vi "Autonomous Independent.vi"   [LabVIEW 2019]
doc: "This VI is called when autonomous begins, and will automatically be terminated when autonomous ends. You can carry out timed or sensor driven robot movement independently without needing to return to the caller."
uses:
  <vilib>/Rock Robotics/WPI/ThirdParty/Phoenix-LabVIEW/Motor Controller/Controls/CTRE_Phoenix_MotorControl_ControlMode.ctl
  <vilib>/Rock Robotics/WPI/Utilities/WPI_GetSetVariantRefNum.vi
  <vilib>/Rock Robotics/Network Tables/NT Read String.vi
  <vilib>/Rock Robotics/Network Tables/NT Write Numeric Array.vi
  <vilib>/Rock Robotics/WPI/RobotDrive/WPI_RobotDriveArcadeDrive_Standard(NoSaturation).vi
panel:
  # "Be sure to right-click and choose Data Operations>>Make Current Value default if you want to save the array values with the VI"
types:
  T1 = typedef "WPI_JoystickDevRef.ctl" = cluster{"Device":T2}
  T2 = typedef "WPI_JoystickDeviceEnum.ctl" = enum16{"USB 0", "USB 1", "USB 2", "USB 3", "USB 4", "USB 5"}
  T3 = typedef "WPI_RobotDriveDevRef.ctl" = cluster{"DevStatus":errorcluster, "Motors[]":T4[], "Square Inputs":bool, "Max Output":dbl}
  T4 = typedef "WPI_MotorControlDeviceRef.ctl" = cluster{"DeviceStatus":errorcluster, "Type":T5, "PWM":cluster{"PWM Channel":T6, "DeadBand":T7}, "CAN":cluster{"Device Number":u8, "SetOutput VI Ref":variant, "GetOutput VI Ref":variant, "Enable VI Ref":variant, "Disable VI Ref":variant, "Data":variant}, "Invert":bool, "DIO PWM":cluster{"PWM \"Enable\" Channel":T6, "DIOChannel":T8, "PWM Rate":dbl}}
  T5 = typedef "WPI_MotorControlType.ctl" = enum16{"PWM", "CAN", "DIO PWM"}
  T6 = typedef "FPGA_DIOPWMChannel.ctl" = enum8{"PWM 0", "PWM 1", "PWM 2", "PWM 3", "PWM 4", "PWM 5", "PWM 6", "PWM 7", "PWM 8", "PWM 9", "PWM MXP 0", "PWM MXP 1", "PWM MXP 2", "PWM MXP 3", "PWM MXP 4", "PWM MXP 5", "PWM MXP 6", "PWM MXP 7", "PWM MXP 8", "PWM MXP 9", "Invalid"}
  T7 = typedef "WPI_PWMDeadband.ctl" = cluster{"Name":string, "maxPositivePwm":i32, "minPositivePwm":i32, "centerPwm":i32, "maxNegativePwm":i32, "minNegativePwm":i32, "angularRange":u16}
  T8 = typedef "FPGA_DIOChannel.ctl" = enum8{"DIO 0", "DIO 1", "DIO 2", "DIO 3", "DIO 4", "DIO 5", "DIO 6", "DIO 7", "DIO 8", "DIO 9", "DIO MXP 0", "DIO MXP 1", "DIO MXP 2", "DIO MXP 3", "DIO MXP 4", "DIO MXP 5", "DIO MXP 6", "DIO MXP 7", "DIO MXP 8", "DIO MXP 9", "DIO MXP 10", "DIO MXP 11", "DIO MXP 12", "DIO MXP 13", "DIO MXP 14", "DIO MXP 15", "SPI Port CS1", "SPI Port CS2", "SPI Port CS3", "SPI Port MISO", "SPI Port MOSI", "Invalid"}
  T9 = typedef "CTRE_Phoenix_MotorControl_ControlMode.ctl" = u16
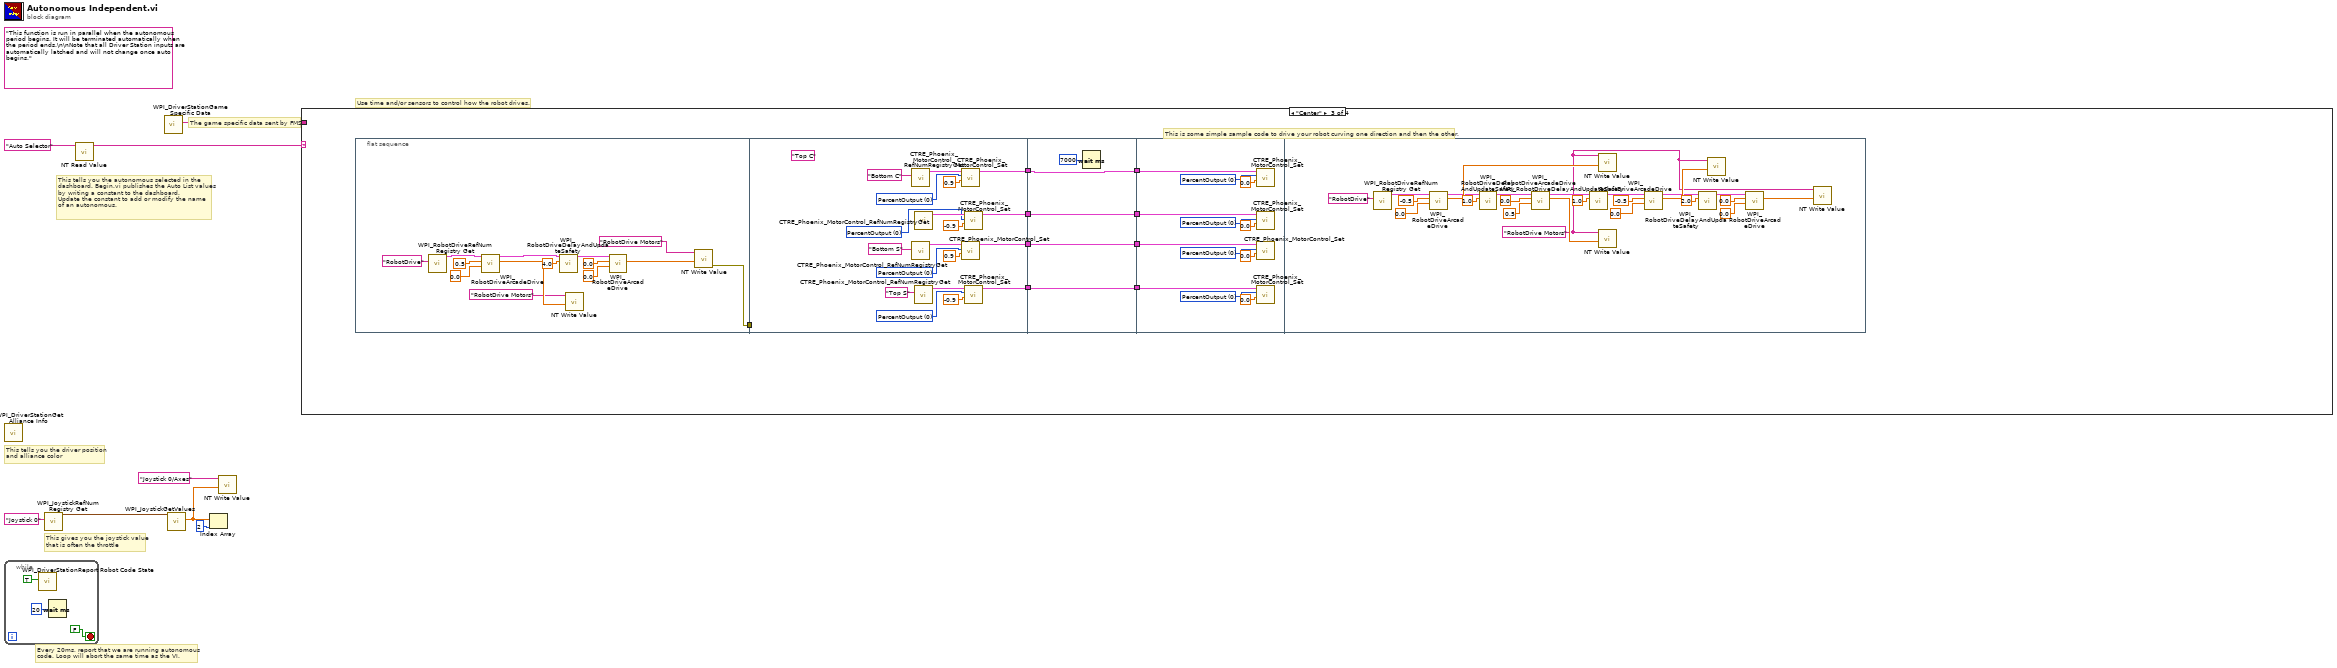
[diagram p0: block diagram]
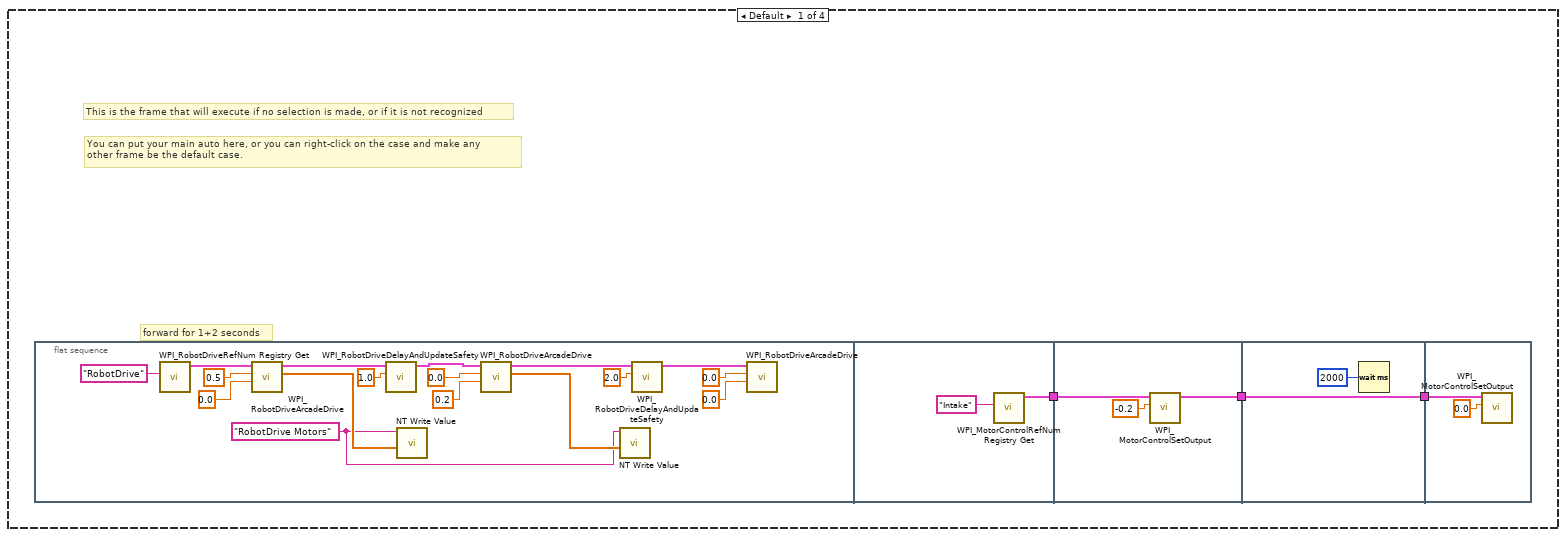
[diagram p2: hidden frame]
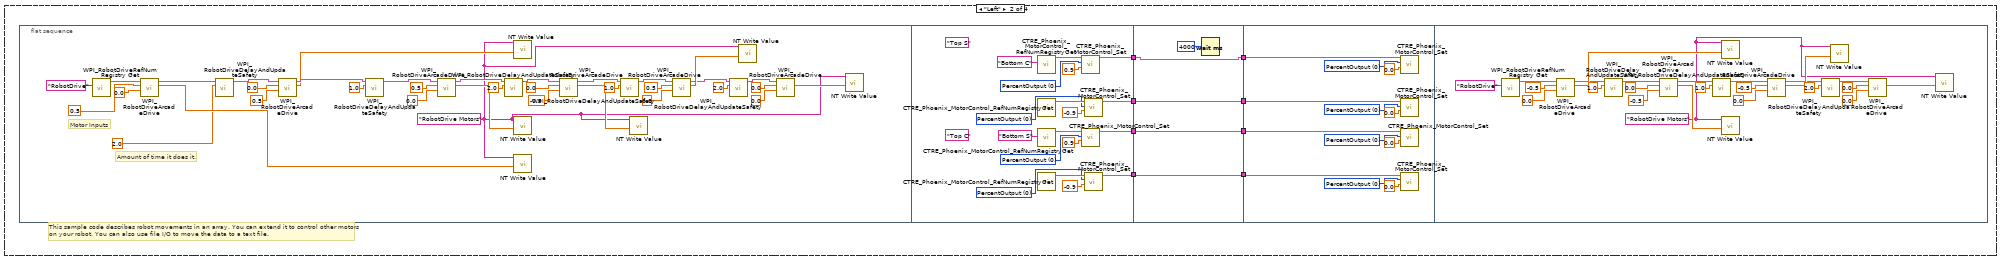
[diagram p3: hidden frame]
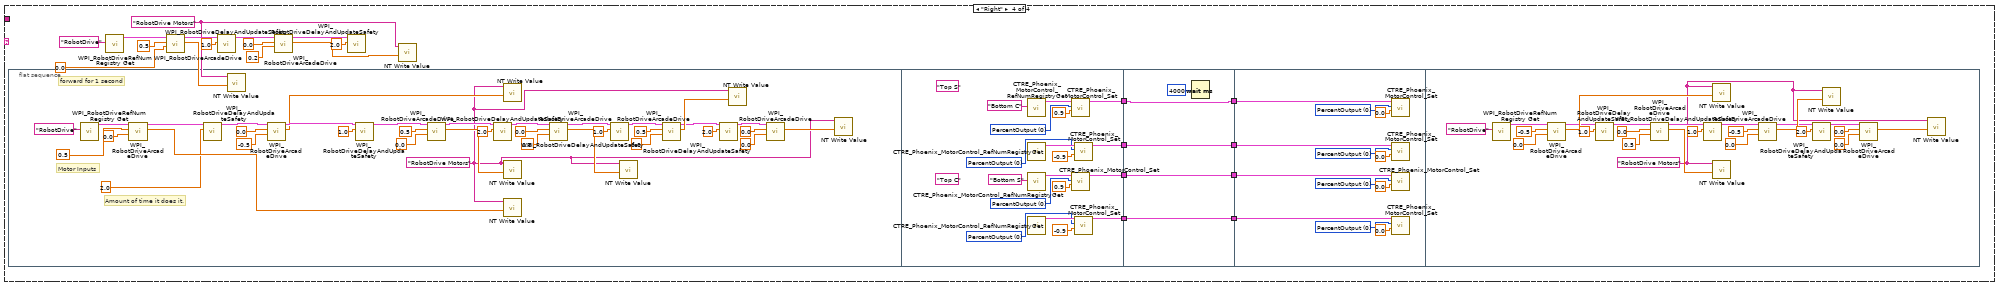
[diagram p4: hidden frame]
diagram:
  (unwired) "This function is run in parallel when the autonomous period begins. It will be terminated automatically when the period ends.\n\nNote that all Driver Station inputs are automatically latched and will not change once auto begins."
  # "The game specific data sent by FMS"
  # "This tells you the autonomous selected in the \ndashboard. Begin.vi publishes the Auto List values\nby writing a constant to the dashboard.\nUpdate the constant to add or modify the name\nof an autonomous."
  # "Every 20ms, report that we are running autonomous\ncode. Loop will abort the same time as the VI."
  # "This gives you the joystick value\nthat is often the throttle"
  # "Use time and/or sensors to control how the robot drives."
  # "This tells you the driver position\nand alliance color"
  n1 = call <vilib>:"WPI_DriverStationGet Alliance Info.vi"() -> ()  [unwired: 12 out]
  n2 = while {
    stop <- FALSE stop-if-true
    n3 = call <vilib>:"WPI_DriverStationReport Robot Code State.vi"("Autonomous"=TRUE) -> ()  [unwired: 10 in, 1 out]
    n4 = Wait (ms)(milliseconds to wait=u32 20) -> ()  [unwired: 1 out]
  }
  n5 = call <vilib>:"WPI_JoystickRefNum Registry Get.vi"("refnum name"="Joystick 0") -> ("JoystickDevRef"=w7:T1)  [unwired: 1 in, 9 out]
  n6 = call-poly <vilib>:"NT Read Value.vi"("Name"="Auto Selector") -> ("String"=w4:string)  [unwired: 9 in, 1 out]
  n7 = call <vilib>:"WPI_DriverStationGame Specific Data.vi"() -> ("Game Specific Data"=w1:string)  [unwired: 11 in]
  n8 = call <vilib>:"WPI_JoystickGetValues.vi"("JoystickDevRef"=w7) -> ("Axes"=w3:dbl[])  [unwired: 6 in, 4 out]
  n9 = Index Array(array=w3, index=2) -> ()  [unwired: 1 out]
  n10 = call-poly <vilib>:"NT Write Value.vi"("Numeric Array"=w3, "Name"="Joystick 0/Axes") -> ()  [unwired: 9 in, 1 out]
  n11 = case shown="\"Center\"" w4 {
    tunnel: w1 -> [_ _ _ _]
    frame Default {
      # "forward for 1+2 seconds"
      # "You can put your main auto here, or you can right-click on the case and make any\nother frame be the default case."
      # "This is the frame that will execute if no selection is made, or if it is not recognized"
      n12 = flat-sequence {
        tunnel: [w32] -> w14
        tunnel: w14 -> [w36]
        tunnel: [w34] -> w13
        tunnel: w13 -> [w37]
        tunnel: [w37] -> w12
        tunnel: w12 -> [w39]
        frame #0 {
          w24 = "RobotDrive Motors" ("Name")
          n13 = call <vilib>:"WPI_RobotDriveRefNum Registry Get.vi"("refnum name"="RobotDrive") -> ("RobotDriveDevRef"=w26:T3)  [unwired: 1 in, 9 out]
          n14 = call-poly <vilib>:"WPI_RobotDriveArcadeDrive.vi"("Y axis value"=0.0 ("X axis value"), "X axis value"=0.5, "RobotDriveDevRef"=w26) -> ("Motor Values"=w28:dbl[], "RobotDriveDevRef"=w27:T3)  [unwired: 1 in, 6 out]
          n15 = call <vilib>:"WPI_RobotDriveDelayAndUpdateSafety.vi"("Delay (s)"=1.0, "RobotDriveDevRef"=w27) -> ("RobotDriveDevRef 2"=w29:T3)  [unwired: 8 in, 1 out]
          n16 = call-poly <vilib>:"NT Write Value.vi"("Numeric Array"=w28, "Name"=w24) -> ()  [unwired: 9 in, 1 out]
          n17 = call-poly <vilib>:"WPI_RobotDriveArcadeDrive.vi"("Y axis value"=0.2, "X axis value"=0.0, "RobotDriveDevRef"=w29) -> ("Motor Values"=w30:dbl[], "RobotDriveDevRef"=w31:T3)  [unwired: 1 in, 6 out]
          n18 = call-poly <vilib>:"NT Write Value.vi"("Numeric Array"=w30, "Name"=w24) -> ()  [unwired: 9 in, 1 out]
          n19 = call <vilib>:"WPI_RobotDriveDelayAndUpdateSafety.vi"("Delay (s)"=2.0, "RobotDriveDevRef"=w31) -> ("RobotDriveDevRef 2"=w17:T3)  [unwired: 8 in, 1 out]
          n20 = call-poly <vilib>:"WPI_RobotDriveArcadeDrive.vi"("Y axis value"=0.0, "X axis value"=0.0, "RobotDriveDevRef"=w17) -> ()  [unwired: 6 in, 3 out]
        }
        frame #1 {
          n21 = call <vilib>:"WPI_MotorControlRefNum Registry Get.vi"("refnum name"="Intake") -> ("MotorControlDevRef"=w32:T4)  [unwired: 9 in, 1 out]
        }
        frame #2 {
          n22 = call <vilib>:"WPI_MotorControlSetOutput.vi"("Output"=-0.2, "MotorControlDevRef"=w36) -> ("MotorControlDevRef"=w34:T4)  [unwired: 7 in, 2 out]
        }
        frame #3 {
          n23 = Wait (ms)(milliseconds to wait=u32 2000) -> ()  [unwired: 1 out]
        }
        frame #4 {
          n24 = call <vilib>:"WPI_MotorControlSetOutput.vi"("Output"=0.0, "MotorControlDevRef"=w39) -> ()  [unwired: 7 in, 3 out]
        }
      }
    }
    frame "Left" {
      # "This sample code describes robot movements in an array. You can extend it to control other motors\non your robot. You can also use file I/O to move the data to a text file."
      n25 = flat-sequence {
        tunnel: [w88] -> w48
        tunnel: [w87] -> w46
        tunnel: [w86] -> w44
        tunnel: [w85] -> w42
        tunnel: w48 -> [w106]
        tunnel: [w106] -> w47
        tunnel: w46 -> [w105]
        tunnel: [w105] -> w45
        tunnel: w44 -> [w104]
        tunnel: [w104] -> w43
        tunnel: w42 -> [w103]
        tunnel: [w103] -> w41
        tunnel: w47 -> [w111]
        tunnel: w45 -> [w110]
        tunnel: w43 -> [w109]
        tunnel: w41 -> [w108]
        frame #0 {
          w49 = "RobotDrive Motors" ("Name")
          # "Amount of time it does it."
          # "Motor Inputs"
          n26 = call <vilib>:"WPI_RobotDriveRefNum Registry Get.vi"("refnum name"="RobotDrive") -> ("RobotDriveDevRef"=w79:T3)  [unwired: 1 in, 9 out]
          n27 = call-poly <vilib>:"WPI_RobotDriveArcadeDrive.vi"("Y axis value"=0.0 ("X axis value"), "X axis value"=0.5, "RobotDriveDevRef"=w79) -> ("Motor Values"=w81:dbl[], "RobotDriveDevRef"=w80:T3)  [unwired: 1 in, 6 out]
          n28 = call <vilib>:"WPI_RobotDriveDelayAndUpdateSafety.vi"("Delay (s)"=2.0, "RobotDriveDevRef"=w80) -> ("RobotDriveDevRef 2"=w82:T3)  [unwired: 8 in, 1 out]
          n29 = call-poly <vilib>:"WPI_RobotDriveArcadeDrive.vi"("Y axis value"=0.5, "X axis value"=0.0, "RobotDriveDevRef"=w82) -> ("Motor Values"=w83:dbl[], "RobotDriveDevRef"=w84:T3)  [unwired: 1 in, 6 out]
          n30 = call <vilib>:"WPI_RobotDriveDelayAndUpdateSafety.vi"("Delay (s)"=1.0, "RobotDriveDevRef"=w84) -> ("RobotDriveDevRef 2"=w68:T3)  [unwired: 8 in, 1 out]
          n31 = call-poly <vilib>:"WPI_RobotDriveArcadeDrive.vi"("Y axis value"=0.0 ("X axis value"), "X axis value"=0.5, "RobotDriveDevRef"=w68) -> ("Motor Values"=w71:dbl[], "RobotDriveDevRef"=w67:T3)  [unwired: 1 in, 6 out]
          n32 = call <vilib>:"WPI_RobotDriveDelayAndUpdateSafety.vi"("Delay (s)"=2.0, "RobotDriveDevRef"=w67) -> ("RobotDriveDevRef 2"=w60:T3)  [unwired: 8 in, 1 out]
          n33 = call-poly <vilib>:"NT Write Value.vi"("Numeric Array"=w83, "Name"=w49) -> ()  [unwired: 9 in, 1 out]
          n34 = call-poly <vilib>:"NT Write Value.vi"("Numeric Array"=w71, "Name"=w49) -> ()  [unwired: 9 in, 1 out]
          n35 = call-poly <vilib>:"NT Write Value.vi"("Numeric Array"=w81, "Name"=w49) -> ()  [unwired: 9 in, 1 out]
          n36 = call-poly <vilib>:"WPI_RobotDriveArcadeDrive.vi"("Y axis value"=-0.5 ("X axis value"), "X axis value"=0.0, "RobotDriveDevRef"=w60) -> ("Motor Values"=w65:dbl[], "RobotDriveDevRef"=w62:T3)  [unwired: 1 in, 6 out]
          n37 = call <vilib>:"WPI_RobotDriveDelayAndUpdateSafety.vi"("Delay (s)"=1.0, "RobotDriveDevRef"=w62) -> ("RobotDriveDevRef 2"=w54:T3)  [unwired: 8 in, 1 out]
          n38 = call-poly <vilib>:"NT Write Value.vi"("Numeric Array"=w65, "Name"=w49) -> ()  [unwired: 9 in, 1 out]
          n39 = call-poly <vilib>:"WPI_RobotDriveArcadeDrive.vi"("Y axis value"=0.0 ("X axis value"), "X axis value"=0.5, "RobotDriveDevRef"=w54) -> ("Motor Values"=w59:dbl[], "RobotDriveDevRef"=w56:T3)  [unwired: 1 in, 6 out]
          n40 = call <vilib>:"WPI_RobotDriveDelayAndUpdateSafety.vi"("Delay (s)"=2.0, "RobotDriveDevRef"=w56) -> ("RobotDriveDevRef 2"=w50:T3)  [unwired: 8 in, 1 out]
          n41 = call-poly <vilib>:"NT Write Value.vi"("Numeric Array"=w59, "Name"=w49) -> ()  [unwired: 9 in, 1 out]
          n42 = call-poly <vilib>:"WPI_RobotDriveArcadeDrive.vi"("Y axis value"=0.0 ("X axis value"), "X axis value"=0.0, "RobotDriveDevRef"=w50) -> ("Motor Values"=w53:dbl[])  [unwired: 1 in, 7 out]
          n43 = call-poly <vilib>:"NT Write Value.vi"("Numeric Array"=w53, "Name"=w49) -> ()  [unwired: 9 in, 1 out]
        }
        frame #1 {
          w90 = T9 0 items=["PercentOutput"=0, "Position"=1, "Velocity"=2, "Current"=3, "Follower"=5, "MotionProfile"=6, "MotionMagic"=7, "MotionProfileArc"=10, "Disabled"=15] ("Control Mode")
          w94 = T9 0 items=["PercentOutput"=0, "Position"=1, "Velocity"=2, "Current"=3, "Follower"=5, "MotionProfile"=6, "MotionMagic"=7, "MotionProfileArc"=10, "Disabled"=15] ("Control Mode")
          (unwired) "Top C" ("refnum name")
          w97 = T9 0 items=["PercentOutput"=0, "Position"=1, "Velocity"=2, "Current"=3, "Follower"=5, "MotionProfile"=6, "MotionMagic"=7, "MotionProfileArc"=10, "Disabled"=15] ("Control Mode")
          w101 = T9 0 items=["PercentOutput"=0, "Position"=1, "Velocity"=2, "Current"=3, "Follower"=5, "MotionProfile"=6, "MotionMagic"=7, "MotionProfileArc"=10, "Disabled"=15] ("Control Mode")
          (unwired) "Top S" ("refnum name")
          n44 = call <vilib>:"CTRE_Phoenix_MotorControl_RefNumRegistryGet.vi"("refnum name"="Bottom C") -> ("PhoenixMotorControlDevRef"=w91:T4)  [unwired: 9 in, 1 out]
          n45 = call <vilib>:"CTRE_Phoenix_MotorControl_RefNumRegistryGet.vi"() -> ("PhoenixMotorControlDevRef"=w95:T4)  [unwired: 10 in, 1 out]
          n46 = call <vilib>:"CTRE_Phoenix_MotorControl_RefNumRegistryGet.vi"("refnum name"="Bottom S") -> ("PhoenixMotorControlDevRef"=w98:T4)  [unwired: 9 in, 1 out]
          n47 = call <vilib>:"CTRE_Phoenix_MotorControl_RefNumRegistryGet.vi"() -> ("PhoenixMotorControlDevRef"=w102:T4)  [unwired: 10 in, 1 out]
          n48 = call <vilib>:"CTRE_Phoenix_MotorControl_Set.vi"("Output"=0.9, "Control Mode"=w90, "PhoenixMotorControlDevRef"=w91) -> ("PhoenixMotorControlDevRef"=w85:T4)  [unwired: 7 in, 1 out]
          n49 = call <vilib>:"CTRE_Phoenix_MotorControl_Set.vi"("Output"=0.9, "Control Mode"=w97, "PhoenixMotorControlDevRef"=w98) -> ("PhoenixMotorControlDevRef"=w87:T4)  [unwired: 7 in, 1 out]
          n50 = call <vilib>:"CTRE_Phoenix_MotorControl_Set.vi"("Output"=-0.9, "Control Mode"=w94, "PhoenixMotorControlDevRef"=w95) -> ("PhoenixMotorControlDevRef"=w86:T4)  [unwired: 7 in, 1 out]
          n51 = call <vilib>:"CTRE_Phoenix_MotorControl_Set.vi"("Output"=-0.9, "Control Mode"=w101, "PhoenixMotorControlDevRef"=w102) -> ("PhoenixMotorControlDevRef"=w88:T4)  [unwired: 7 in, 1 out]
        }
        frame #2 {
          n52 = Wait (ms)(milliseconds to wait=u32 4000) -> ()  [unwired: 1 out]
        }
        frame #3 {
          w113 = T9 0 items=["PercentOutput"=0, "Position"=1, "Velocity"=2, "Current"=3, "Follower"=5, "MotionProfile"=6, "MotionMagic"=7, "MotionProfileArc"=10, "Disabled"=15] ("Control Mode")
          w115 = T9 0 items=["PercentOutput"=0, "Position"=1, "Velocity"=2, "Current"=3, "Follower"=5, "MotionProfile"=6, "MotionMagic"=7, "MotionProfileArc"=10, "Disabled"=15] ("Control Mode")
          w117 = T9 0 items=["PercentOutput"=0, "Position"=1, "Velocity"=2, "Current"=3, "Follower"=5, "MotionProfile"=6, "MotionMagic"=7, "MotionProfileArc"=10, "Disabled"=15] ("Control Mode")
          w119 = T9 0 items=["PercentOutput"=0, "Position"=1, "Velocity"=2, "Current"=3, "Follower"=5, "MotionProfile"=6, "MotionMagic"=7, "MotionProfileArc"=10, "Disabled"=15] ("Control Mode")
          n53 = call <vilib>:"CTRE_Phoenix_MotorControl_Set.vi"("Output"=0.0, "Control Mode"=w113, "PhoenixMotorControlDevRef"=w108) -> ()  [unwired: 7 in, 2 out]
          n54 = call <vilib>:"CTRE_Phoenix_MotorControl_Set.vi"("Output"=0.0, "Control Mode"=w115, "PhoenixMotorControlDevRef"=w109) -> ()  [unwired: 7 in, 2 out]
          n55 = call <vilib>:"CTRE_Phoenix_MotorControl_Set.vi"("Output"=0.0, "Control Mode"=w117, "PhoenixMotorControlDevRef"=w110) -> ()  [unwired: 7 in, 2 out]
          n56 = call <vilib>:"CTRE_Phoenix_MotorControl_Set.vi"("Output"=0.0, "Control Mode"=w119, "PhoenixMotorControlDevRef"=w111) -> ()  [unwired: 7 in, 2 out]
        }
        frame #4 {
          w120 = "RobotDrive Motors" ("Name")
          n57 = call <vilib>:"WPI_RobotDriveRefNum Registry Get.vi"("refnum name"="RobotDrive") -> ("RobotDriveDevRef"=w141:T3)  [unwired: 1 in, 9 out]
          n58 = call-poly <vilib>:"WPI_RobotDriveArcadeDrive.vi"("Y axis value"=0.0 ("X axis value"), "X axis value"=-0.5, "RobotDriveDevRef"=w141) -> ("Motor Values"=w143:dbl[], "RobotDriveDevRef"=w142:T3)  [unwired: 1 in, 6 out]
          n59 = call <vilib>:"WPI_RobotDriveDelayAndUpdateSafety.vi"("Delay (s)"=1.0, "RobotDriveDevRef"=w142) -> ("RobotDriveDevRef 2"=w131:T3)  [unwired: 8 in, 1 out]
          n60 = call-poly <vilib>:"WPI_RobotDriveArcadeDrive.vi"("Y axis value"=-0.5 ("X axis value"), "X axis value"=0.0, "RobotDriveDevRef"=w131) -> ("Motor Values"=w136:dbl[], "RobotDriveDevRef"=w135:T3)  [unwired: 1 in, 6 out]
          n61 = call <vilib>:"WPI_RobotDriveDelayAndUpdateSafety.vi"("Delay (s)"=1.0, "RobotDriveDevRef"=w135) -> ("RobotDriveDevRef 2"=w125:T3)  [unwired: 8 in, 1 out]
          n62 = call-poly <vilib>:"NT Write Value.vi"("Numeric Array"=w143, "Name"=w120) -> ()  [unwired: 9 in, 1 out]
          n63 = call-poly <vilib>:"NT Write Value.vi"("Numeric Array"=w136, "Name"=w120) -> ()  [unwired: 9 in, 1 out]
          n64 = call-poly <vilib>:"WPI_RobotDriveArcadeDrive.vi"("Y axis value"=0.0 ("X axis value"), "X axis value"=-0.5, "RobotDriveDevRef"=w125) -> ("Motor Values"=w130:dbl[], "RobotDriveDevRef"=w129:T3)  [unwired: 1 in, 6 out]
          n65 = call <vilib>:"WPI_RobotDriveDelayAndUpdateSafety.vi"("Delay (s)"=2.0, "RobotDriveDevRef"=w129) -> ("RobotDriveDevRef 2"=w121:T3)  [unwired: 8 in, 1 out]
          n66 = call-poly <vilib>:"NT Write Value.vi"("Numeric Array"=w130, "Name"=w120) -> ()  [unwired: 9 in, 1 out]
          n67 = call-poly <vilib>:"WPI_RobotDriveArcadeDrive.vi"("Y axis value"=0.0 ("X axis value"), "X axis value"=0.0, "RobotDriveDevRef"=w121) -> ("Motor Values"=w124:dbl[])  [unwired: 1 in, 7 out]
          n68 = call-poly <vilib>:"NT Write Value.vi"("Numeric Array"=w124, "Name"=w120) -> ()  [unwired: 9 in, 1 out]
        }
      }
    }
    frame "Center" {
      # "This is some simple sample code to drive your robot curving one direction and then the other."
      n69 = flat-sequence {
        tunnel: [w153] -> w152
        tunnel: w152 -> [_]
        tunnel: [w170] -> w151
        tunnel: [w169] -> w148
        tunnel: [w168] -> w147
        tunnel: [w167] -> w144
        tunnel: w151 -> [w189]
        tunnel: [w189] -> w150
        tunnel: [w188] -> w149
        tunnel: w148 -> [w188]
        tunnel: w147 -> [w187]
        tunnel: [w187] -> w146
        tunnel: [w186] -> w145
        tunnel: w144 -> [w186]
        tunnel: w150 -> [w194]
        tunnel: w149 -> [w193]
        tunnel: w146 -> [w192]
        tunnel: w145 -> [w191]
        frame #0 {
          n70 = call <vilib>:"WPI_RobotDriveRefNum Registry Get.vi"("refnum name"="RobotDrive") -> ("RobotDriveDevRef"=w164:T3)  [unwired: 1 in, 9 out]
          n71 = call-poly <vilib>:"WPI_RobotDriveArcadeDrive.vi"("Y axis value"=0.0 ("X axis value"), "X axis value"=0.5, "RobotDriveDevRef"=w164) -> ("Motor Values"=w166:dbl[], "RobotDriveDevRef"=w165:T3)  [unwired: 1 in, 6 out]
          n72 = call <vilib>:"WPI_RobotDriveDelayAndUpdateSafety.vi"("Delay (s)"=4.0, "RobotDriveDevRef"=w165) -> ("RobotDriveDevRef 2"=w154:T3)  [unwired: 8 in, 1 out]
          n73 = call-poly <vilib>:"NT Write Value.vi"("Numeric Array"=w166, "Name"="RobotDrive Motors") -> ()  [unwired: 9 in, 1 out]
          n74 = call-poly <vilib>:"WPI_RobotDriveArcadeDrive.vi"("Y axis value"=0.0 ("X axis value"), "X axis value"=0.0, "RobotDriveDevRef"=w154) -> ("Motor Values"=w158:dbl[])  [unwired: 1 in, 7 out]
          n75 = call-poly <vilib>:"NT Write Value.vi"("Numeric Array"=w158, "Name"="RobotDrive Motors") -> ("error out"=w153:errorcluster)  [unwired: 9 in]
        }
        frame #1 {
          w172 = T9 0 items=["PercentOutput"=0, "Position"=1, "Velocity"=2, "Current"=3, "Follower"=5, "MotionProfile"=6, "MotionMagic"=7, "MotionProfileArc"=10, "Disabled"=15] ("Control Mode")
          w176 = T9 0 items=["PercentOutput"=0, "Position"=1, "Velocity"=2, "Current"=3, "Follower"=5, "MotionProfile"=6, "MotionMagic"=7, "MotionProfileArc"=10, "Disabled"=15] ("Control Mode")
          (unwired) "Top C" ("refnum name")
          w179 = T9 0 items=["PercentOutput"=0, "Position"=1, "Velocity"=2, "Current"=3, "Follower"=5, "MotionProfile"=6, "MotionMagic"=7, "MotionProfileArc"=10, "Disabled"=15] ("Control Mode")
          w183 = T9 0 items=["PercentOutput"=0, "Position"=1, "Velocity"=2, "Current"=3, "Follower"=5, "MotionProfile"=6, "MotionMagic"=7, "MotionProfileArc"=10, "Disabled"=15] ("Control Mode")
          n76 = call <vilib>:"CTRE_Phoenix_MotorControl_RefNumRegistryGet.vi"("refnum name"="Bottom C") -> ("PhoenixMotorControlDevRef"=w173:T4)  [unwired: 9 in, 1 out]
          n77 = call <vilib>:"CTRE_Phoenix_MotorControl_RefNumRegistryGet.vi"("refnum name"="Bottom S") -> ("PhoenixMotorControlDevRef"=w180:T4)  [unwired: 9 in, 1 out]
          n78 = call <vilib>:"CTRE_Phoenix_MotorControl_RefNumRegistryGet.vi"() -> ("PhoenixMotorControlDevRef"=w177:T4)  [unwired: 10 in, 1 out]
          n79 = call <vilib>:"CTRE_Phoenix_MotorControl_RefNumRegistryGet.vi"("refnum name"="Top S") -> ("PhoenixMotorControlDevRef"=w184:T4)  [unwired: 9 in, 1 out]
          n80 = call <vilib>:"CTRE_Phoenix_MotorControl_Set.vi"("Output"=0.9, "Control Mode"=w172, "PhoenixMotorControlDevRef"=w173) -> ("PhoenixMotorControlDevRef"=w167:T4)  [unwired: 7 in, 1 out]
          n81 = call <vilib>:"CTRE_Phoenix_MotorControl_Set.vi"("Output"=0.9, "Control Mode"=w179, "PhoenixMotorControlDevRef"=w180) -> ("PhoenixMotorControlDevRef"=w169:T4)  [unwired: 7 in, 1 out]
          n82 = call <vilib>:"CTRE_Phoenix_MotorControl_Set.vi"("Output"=-0.9, "Control Mode"=w176, "PhoenixMotorControlDevRef"=w177) -> ("PhoenixMotorControlDevRef"=w168:T4)  [unwired: 7 in, 1 out]
          n83 = call <vilib>:"CTRE_Phoenix_MotorControl_Set.vi"("Output"=-0.9, "Control Mode"=w183, "PhoenixMotorControlDevRef"=w184) -> ("PhoenixMotorControlDevRef"=w170:T4)  [unwired: 7 in, 1 out]
        }
        frame #2 {
          n84 = Wait (ms)(milliseconds to wait=u32 7000) -> ()  [unwired: 1 out]
        }
        frame #3 {
          w196 = T9 0 items=["PercentOutput"=0, "Position"=1, "Velocity"=2, "Current"=3, "Follower"=5, "MotionProfile"=6, "MotionMagic"=7, "MotionProfileArc"=10, "Disabled"=15] ("Control Mode")
          w198 = T9 0 items=["PercentOutput"=0, "Position"=1, "Velocity"=2, "Current"=3, "Follower"=5, "MotionProfile"=6, "MotionMagic"=7, "MotionProfileArc"=10, "Disabled"=15] ("Control Mode")
          w200 = T9 0 items=["PercentOutput"=0, "Position"=1, "Velocity"=2, "Current"=3, "Follower"=5, "MotionProfile"=6, "MotionMagic"=7, "MotionProfileArc"=10, "Disabled"=15] ("Control Mode")
          w202 = T9 0 items=["PercentOutput"=0, "Position"=1, "Velocity"=2, "Current"=3, "Follower"=5, "MotionProfile"=6, "MotionMagic"=7, "MotionProfileArc"=10, "Disabled"=15] ("Control Mode")
          n85 = call <vilib>:"CTRE_Phoenix_MotorControl_Set.vi"("Output"=0.0, "Control Mode"=w196, "PhoenixMotorControlDevRef"=w191) -> ()  [unwired: 7 in, 2 out]
          n86 = call <vilib>:"CTRE_Phoenix_MotorControl_Set.vi"("Output"=0.0, "Control Mode"=w198, "PhoenixMotorControlDevRef"=w192) -> ()  [unwired: 7 in, 2 out]
          n87 = call <vilib>:"CTRE_Phoenix_MotorControl_Set.vi"("Output"=0.0, "Control Mode"=w200, "PhoenixMotorControlDevRef"=w193) -> ()  [unwired: 7 in, 2 out]
          n88 = call <vilib>:"CTRE_Phoenix_MotorControl_Set.vi"("Output"=0.0, "Control Mode"=w202, "PhoenixMotorControlDevRef"=w194) -> ()  [unwired: 7 in, 2 out]
        }
        frame #4 {
          w203 = "RobotDrive Motors" ("Name")
          n89 = call <vilib>:"WPI_RobotDriveRefNum Registry Get.vi"("refnum name"="RobotDrive") -> ("RobotDriveDevRef"=w224:T3)  [unwired: 1 in, 9 out]
          n90 = call-poly <vilib>:"WPI_RobotDriveArcadeDrive.vi"("Y axis value"=0.0 ("X axis value"), "X axis value"=-0.5, "RobotDriveDevRef"=w224) -> ("Motor Values"=w226:dbl[], "RobotDriveDevRef"=w225:T3)  [unwired: 1 in, 6 out]
          n91 = call <vilib>:"WPI_RobotDriveDelayAndUpdateSafety.vi"("Delay (s)"=1.0, "RobotDriveDevRef"=w225) -> ("RobotDriveDevRef 2"=w214:T3)  [unwired: 8 in, 1 out]
          n92 = call-poly <vilib>:"WPI_RobotDriveArcadeDrive.vi"("Y axis value"=0.5 ("X axis value"), "X axis value"=0.0, "RobotDriveDevRef"=w214) -> ("Motor Values"=w219:dbl[], "RobotDriveDevRef"=w218:T3)  [unwired: 1 in, 6 out]
          n93 = call <vilib>:"WPI_RobotDriveDelayAndUpdateSafety.vi"("Delay (s)"=1.0, "RobotDriveDevRef"=w218) -> ("RobotDriveDevRef 2"=w208:T3)  [unwired: 8 in, 1 out]
          n94 = call-poly <vilib>:"NT Write Value.vi"("Numeric Array"=w226, "Name"=w203) -> ()  [unwired: 9 in, 1 out]
          n95 = call-poly <vilib>:"NT Write Value.vi"("Numeric Array"=w219, "Name"=w203) -> ()  [unwired: 9 in, 1 out]
          n96 = call-poly <vilib>:"WPI_RobotDriveArcadeDrive.vi"("Y axis value"=0.0 ("X axis value"), "X axis value"=-0.5, "RobotDriveDevRef"=w208) -> ("Motor Values"=w213:dbl[], "RobotDriveDevRef"=w212:T3)  [unwired: 1 in, 6 out]
          n97 = call <vilib>:"WPI_RobotDriveDelayAndUpdateSafety.vi"("Delay (s)"=2.0, "RobotDriveDevRef"=w212) -> ("RobotDriveDevRef 2"=w204:T3)  [unwired: 8 in, 1 out]
          n98 = call-poly <vilib>:"NT Write Value.vi"("Numeric Array"=w213, "Name"=w203) -> ()  [unwired: 9 in, 1 out]
          n99 = call-poly <vilib>:"WPI_RobotDriveArcadeDrive.vi"("Y axis value"=0.0 ("X axis value"), "X axis value"=0.0, "RobotDriveDevRef"=w204) -> ("Motor Values"=w207:dbl[])  [unwired: 1 in, 7 out]
          n100 = call-poly <vilib>:"NT Write Value.vi"("Numeric Array"=w207, "Name"=w203) -> ()  [unwired: 9 in, 1 out]
        }
      }
    }
    frame "Right" {
      w239 = "RobotDrive Motors" ("Name")
      # "forward for 1 second"
      n101 = flat-sequence {
        tunnel: [w288] -> w234
        tunnel: [w287] -> w233
        tunnel: [w286] -> w232
        tunnel: [w285] -> w231
        tunnel: w234 -> [w306]
        tunnel: [w306] -> w230
        tunnel: w233 -> [w305]
        tunnel: [w305] -> w229
        tunnel: w232 -> [w304]
        tunnel: [w304] -> w228
        tunnel: w231 -> [w303]
        tunnel: [w303] -> w227
        tunnel: w230 -> [w311]
        tunnel: w229 -> [w310]
        tunnel: w228 -> [w309]
        tunnel: w227 -> [w308]
        frame #0 {
          w249 = "RobotDrive Motors" ("Name")
          # "Amount of time it does it."
          # "Motor Inputs"
          n102 = call <vilib>:"WPI_RobotDriveRefNum Registry Get.vi"("refnum name"="RobotDrive") -> ("RobotDriveDevRef"=w279:T3)  [unwired: 1 in, 9 out]
          n103 = call-poly <vilib>:"WPI_RobotDriveArcadeDrive.vi"("Y axis value"=0.0 ("X axis value"), "X axis value"=0.5, "RobotDriveDevRef"=w279) -> ("Motor Values"=w281:dbl[], "RobotDriveDevRef"=w280:T3)  [unwired: 1 in, 6 out]
          n104 = call <vilib>:"WPI_RobotDriveDelayAndUpdateSafety.vi"("Delay (s)"=2.0, "RobotDriveDevRef"=w280) -> ("RobotDriveDevRef 2"=w282:T3)  [unwired: 8 in, 1 out]
          n105 = call-poly <vilib>:"WPI_RobotDriveArcadeDrive.vi"("Y axis value"=-0.5, "X axis value"=0.0, "RobotDriveDevRef"=w282) -> ("Motor Values"=w283:dbl[], "RobotDriveDevRef"=w284:T3)  [unwired: 1 in, 6 out]
          n106 = call <vilib>:"WPI_RobotDriveDelayAndUpdateSafety.vi"("Delay (s)"=1.0, "RobotDriveDevRef"=w284) -> ("RobotDriveDevRef 2"=w268:T3)  [unwired: 8 in, 1 out]
          n107 = call-poly <vilib>:"WPI_RobotDriveArcadeDrive.vi"("Y axis value"=0.0 ("X axis value"), "X axis value"=0.5, "RobotDriveDevRef"=w268) -> ("Motor Values"=w271:dbl[], "RobotDriveDevRef"=w267:T3)  [unwired: 1 in, 6 out]
          n108 = call <vilib>:"WPI_RobotDriveDelayAndUpdateSafety.vi"("Delay (s)"=2.0, "RobotDriveDevRef"=w267) -> ("RobotDriveDevRef 2"=w260:T3)  [unwired: 8 in, 1 out]
          n109 = call-poly <vilib>:"NT Write Value.vi"("Numeric Array"=w283, "Name"=w249) -> ()  [unwired: 9 in, 1 out]
          n110 = call-poly <vilib>:"NT Write Value.vi"("Numeric Array"=w271, "Name"=w249) -> ()  [unwired: 9 in, 1 out]
          n111 = call-poly <vilib>:"NT Write Value.vi"("Numeric Array"=w281, "Name"=w249) -> ()  [unwired: 9 in, 1 out]
          n112 = call-poly <vilib>:"WPI_RobotDriveArcadeDrive.vi"("Y axis value"=0.5 ("X axis value"), "X axis value"=0.0, "RobotDriveDevRef"=w260) -> ("Motor Values"=w265:dbl[], "RobotDriveDevRef"=w262:T3)  [unwired: 1 in, 6 out]
          n113 = call <vilib>:"WPI_RobotDriveDelayAndUpdateSafety.vi"("Delay (s)"=1.0, "RobotDriveDevRef"=w262) -> ("RobotDriveDevRef 2"=w254:T3)  [unwired: 8 in, 1 out]
          n114 = call-poly <vilib>:"NT Write Value.vi"("Numeric Array"=w265, "Name"=w249) -> ()  [unwired: 9 in, 1 out]
          n115 = call-poly <vilib>:"WPI_RobotDriveArcadeDrive.vi"("Y axis value"=0.0 ("X axis value"), "X axis value"=0.5, "RobotDriveDevRef"=w254) -> ("Motor Values"=w259:dbl[], "RobotDriveDevRef"=w256:T3)  [unwired: 1 in, 6 out]
          n116 = call <vilib>:"WPI_RobotDriveDelayAndUpdateSafety.vi"("Delay (s)"=2.0, "RobotDriveDevRef"=w256) -> ("RobotDriveDevRef 2"=w250:T3)  [unwired: 8 in, 1 out]
          n117 = call-poly <vilib>:"NT Write Value.vi"("Numeric Array"=w259, "Name"=w249) -> ()  [unwired: 9 in, 1 out]
          n118 = call-poly <vilib>:"WPI_RobotDriveArcadeDrive.vi"("Y axis value"=0.0 ("X axis value"), "X axis value"=0.0, "RobotDriveDevRef"=w250) -> ("Motor Values"=w253:dbl[])  [unwired: 1 in, 7 out]
          n119 = call-poly <vilib>:"NT Write Value.vi"("Numeric Array"=w253, "Name"=w249) -> ()  [unwired: 9 in, 1 out]
        }
        frame #1 {
          w290 = T9 0 items=["PercentOutput"=0, "Position"=1, "Velocity"=2, "Current"=3, "Follower"=5, "MotionProfile"=6, "MotionMagic"=7, "MotionProfileArc"=10, "Disabled"=15] ("Control Mode")
          w294 = T9 0 items=["PercentOutput"=0, "Position"=1, "Velocity"=2, "Current"=3, "Follower"=5, "MotionProfile"=6, "MotionMagic"=7, "MotionProfileArc"=10, "Disabled"=15] ("Control Mode")
          (unwired) "Top C" ("refnum name")
          w297 = T9 0 items=["PercentOutput"=0, "Position"=1, "Velocity"=2, "Current"=3, "Follower"=5, "MotionProfile"=6, "MotionMagic"=7, "MotionProfileArc"=10, "Disabled"=15] ("Control Mode")
          w301 = T9 0 items=["PercentOutput"=0, "Position"=1, "Velocity"=2, "Current"=3, "Follower"=5, "MotionProfile"=6, "MotionMagic"=7, "MotionProfileArc"=10, "Disabled"=15] ("Control Mode")
          (unwired) "Top S" ("refnum name")
          n120 = call <vilib>:"CTRE_Phoenix_MotorControl_RefNumRegistryGet.vi"("refnum name"="Bottom C") -> ("PhoenixMotorControlDevRef"=w291:T4)  [unwired: 9 in, 1 out]
          n121 = call <vilib>:"CTRE_Phoenix_MotorControl_RefNumRegistryGet.vi"() -> ("PhoenixMotorControlDevRef"=w295:T4)  [unwired: 10 in, 1 out]
          n122 = call <vilib>:"CTRE_Phoenix_MotorControl_RefNumRegistryGet.vi"("refnum name"="Bottom S") -> ("PhoenixMotorControlDevRef"=w298:T4)  [unwired: 9 in, 1 out]
          n123 = call <vilib>:"CTRE_Phoenix_MotorControl_RefNumRegistryGet.vi"() -> ("PhoenixMotorControlDevRef"=w302:T4)  [unwired: 10 in, 1 out]
          n124 = call <vilib>:"CTRE_Phoenix_MotorControl_Set.vi"("Output"=0.9, "Control Mode"=w290, "PhoenixMotorControlDevRef"=w291) -> ("PhoenixMotorControlDevRef"=w285:T4)  [unwired: 7 in, 1 out]
          n125 = call <vilib>:"CTRE_Phoenix_MotorControl_Set.vi"("Output"=0.9, "Control Mode"=w297, "PhoenixMotorControlDevRef"=w298) -> ("PhoenixMotorControlDevRef"=w287:T4)  [unwired: 7 in, 1 out]
          n126 = call <vilib>:"CTRE_Phoenix_MotorControl_Set.vi"("Output"=-0.9, "Control Mode"=w294, "PhoenixMotorControlDevRef"=w295) -> ("PhoenixMotorControlDevRef"=w286:T4)  [unwired: 7 in, 1 out]
          n127 = call <vilib>:"CTRE_Phoenix_MotorControl_Set.vi"("Output"=-0.9, "Control Mode"=w301, "PhoenixMotorControlDevRef"=w302) -> ("PhoenixMotorControlDevRef"=w288:T4)  [unwired: 7 in, 1 out]
        }
        frame #2 {
          n128 = Wait (ms)(milliseconds to wait=u32 4000) -> ()  [unwired: 1 out]
        }
        frame #3 {
          w313 = T9 0 items=["PercentOutput"=0, "Position"=1, "Velocity"=2, "Current"=3, "Follower"=5, "MotionProfile"=6, "MotionMagic"=7, "MotionProfileArc"=10, "Disabled"=15] ("Control Mode")
          w315 = T9 0 items=["PercentOutput"=0, "Position"=1, "Velocity"=2, "Current"=3, "Follower"=5, "MotionProfile"=6, "MotionMagic"=7, "MotionProfileArc"=10, "Disabled"=15] ("Control Mode")
          w317 = T9 0 items=["PercentOutput"=0, "Position"=1, "Velocity"=2, "Current"=3, "Follower"=5, "MotionProfile"=6, "MotionMagic"=7, "MotionProfileArc"=10, "Disabled"=15] ("Control Mode")
          w319 = T9 0 items=["PercentOutput"=0, "Position"=1, "Velocity"=2, "Current"=3, "Follower"=5, "MotionProfile"=6, "MotionMagic"=7, "MotionProfileArc"=10, "Disabled"=15] ("Control Mode")
          n129 = call <vilib>:"CTRE_Phoenix_MotorControl_Set.vi"("Output"=0.0, "Control Mode"=w313, "PhoenixMotorControlDevRef"=w308) -> ()  [unwired: 7 in, 2 out]
          n130 = call <vilib>:"CTRE_Phoenix_MotorControl_Set.vi"("Output"=0.0, "Control Mode"=w315, "PhoenixMotorControlDevRef"=w309) -> ()  [unwired: 7 in, 2 out]
          n131 = call <vilib>:"CTRE_Phoenix_MotorControl_Set.vi"("Output"=0.0, "Control Mode"=w317, "PhoenixMotorControlDevRef"=w310) -> ()  [unwired: 7 in, 2 out]
          n132 = call <vilib>:"CTRE_Phoenix_MotorControl_Set.vi"("Output"=0.0, "Control Mode"=w319, "PhoenixMotorControlDevRef"=w311) -> ()  [unwired: 7 in, 2 out]
        }
        frame #4 {
          w320 = "RobotDrive Motors" ("Name")
          n133 = call <vilib>:"WPI_RobotDriveRefNum Registry Get.vi"("refnum name"="RobotDrive") -> ("RobotDriveDevRef"=w341:T3)  [unwired: 1 in, 9 out]
          n134 = call-poly <vilib>:"WPI_RobotDriveArcadeDrive.vi"("Y axis value"=0.0 ("X axis value"), "X axis value"=-0.5, "RobotDriveDevRef"=w341) -> ("Motor Values"=w343:dbl[], "RobotDriveDevRef"=w342:T3)  [unwired: 1 in, 6 out]
          n135 = call <vilib>:"WPI_RobotDriveDelayAndUpdateSafety.vi"("Delay (s)"=1.0, "RobotDriveDevRef"=w342) -> ("RobotDriveDevRef 2"=w331:T3)  [unwired: 8 in, 1 out]
          n136 = call-poly <vilib>:"WPI_RobotDriveArcadeDrive.vi"("Y axis value"=0.5 ("X axis value"), "X axis value"=0.0, "RobotDriveDevRef"=w331) -> ("Motor Values"=w336:dbl[], "RobotDriveDevRef"=w335:T3)  [unwired: 1 in, 6 out]
          n137 = call <vilib>:"WPI_RobotDriveDelayAndUpdateSafety.vi"("Delay (s)"=1.0, "RobotDriveDevRef"=w335) -> ("RobotDriveDevRef 2"=w325:T3)  [unwired: 8 in, 1 out]
          n138 = call-poly <vilib>:"NT Write Value.vi"("Numeric Array"=w343, "Name"=w320) -> ()  [unwired: 9 in, 1 out]
          n139 = call-poly <vilib>:"NT Write Value.vi"("Numeric Array"=w336, "Name"=w320) -> ()  [unwired: 9 in, 1 out]
          n140 = call-poly <vilib>:"WPI_RobotDriveArcadeDrive.vi"("Y axis value"=0.0 ("X axis value"), "X axis value"=-0.5, "RobotDriveDevRef"=w325) -> ("Motor Values"=w330:dbl[], "RobotDriveDevRef"=w329:T3)  [unwired: 1 in, 6 out]
          n141 = call <vilib>:"WPI_RobotDriveDelayAndUpdateSafety.vi"("Delay (s)"=2.0, "RobotDriveDevRef"=w329) -> ("RobotDriveDevRef 2"=w321:T3)  [unwired: 8 in, 1 out]
          n142 = call-poly <vilib>:"NT Write Value.vi"("Numeric Array"=w330, "Name"=w320) -> ()  [unwired: 9 in, 1 out]
          n143 = call-poly <vilib>:"WPI_RobotDriveArcadeDrive.vi"("Y axis value"=0.0 ("X axis value"), "X axis value"=0.0, "RobotDriveDevRef"=w321) -> ("Motor Values"=w324:dbl[])  [unwired: 1 in, 7 out]
          n144 = call-poly <vilib>:"NT Write Value.vi"("Numeric Array"=w324, "Name"=w320) -> ()  [unwired: 9 in, 1 out]
        }
      }
      n145 = call <vilib>:"WPI_RobotDriveRefNum Registry Get.vi"("refnum name"="RobotDrive") -> ("RobotDriveDevRef"=w248:T3)  [unwired: 1 in, 9 out]
      n146 = call-poly <vilib>:"WPI_RobotDriveArcadeDrive.vi"("Y axis value"=0.0 ("X axis value"), "X axis value"=0.5, "RobotDriveDevRef"=w248) -> ("Motor Values"=w242:dbl[], "RobotDriveDevRef"=w245:T3)  [unwired: 1 in, 6 out]
      n147 = call <vilib>:"WPI_RobotDriveDelayAndUpdateSafety.vi"("Delay (s)"=1.0, "RobotDriveDevRef"=w245) -> ("RobotDriveDevRef 2"=w241:T3)  [unwired: 8 in, 1 out]
      n148 = call-poly <vilib>:"NT Write Value.vi"("Numeric Array"=w242, "Name"=w239) -> ()  [unwired: 9 in, 1 out]
      n149 = call-poly <vilib>:"WPI_RobotDriveArcadeDrive.vi"("Y axis value"=0.2, "X axis value"=0.0, "RobotDriveDevRef"=w241) -> ("Motor Values"=w240:dbl[], "RobotDriveDevRef"=w238:T3)  [unwired: 1 in, 6 out]
      n150 = call <vilib>:"WPI_RobotDriveDelayAndUpdateSafety.vi"("Delay (s)"=2.0, "RobotDriveDevRef"=w238) -> ()  [unwired: 8 in, 2 out]
      n151 = call-poly <vilib>:"NT Write Value.vi"("Numeric Array"=w240, "Name"=w239) -> ()  [unwired: 9 in, 1 out]
    }
  }
